vi "Close.vi"(8 "error in (no error)":errorcluster, 11 "NIScope in":refnum<class "NIScope.lvclass">) -> (0 "error out":errorcluster, 3 "NIScope out":refnum<class "NIScope.lvclass">)   [LabVIEW 2018, in "ScopePlugins.lvlib" / "NIScope.lvclass"]
doc: "Closes the connection to the scope instrument."
uses:
  NIScope.lvclass
  C:/Users/ico/Documents/Projects/NistPluggableModules/Scope/ScopePlugins/ScopePluginBaseClass/ScopePluginsBase.lvclass
  ScopePluginBaseClass/ScopePluginsBase.lvclass/ScopePluginsBase.ctl
  ScopePluginBaseClass/Accessors/Read Channels.vi
  ScopePluginBaseClass/Accessors/Write Channels.vi
  ScopePluginBaseClass/ScopePluginsBase.lvclass
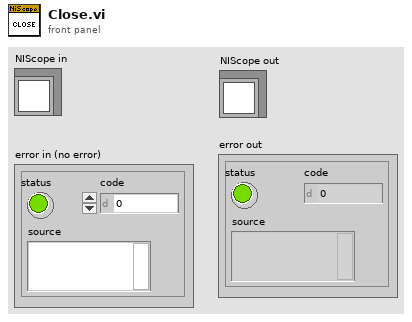
[diagram p1: front panel]
types:
  T1 = typedef "ScopePlugins.lvlib/ScopePluginsBase.lvclass/ChannelSetting(s).ctl" = cluster{"Number of Channels":i32, "Channel(s)":cluster{"Enabled":bool, "Instrument Handle":string, "Channel Name":string, "Maximum Input Frequency":dbl, "Verticle Settings":cluster{"Vertical Range":dbl, "Vertical Offset":dbl, "Probe Attenuation":dbl, "Vertical Coupling":i32}, "Connected":bool, "Input Impedance":dbl}[]}
  T2 = cluster{"Enabled":bool, "Instrument Handle":string, "Channel Name":string, "Maximum Input Frequency":dbl, "Verticle Settings":cluster{"Vertical Range":dbl, "Vertical Offset":dbl, "Probe Attenuation":dbl, "Vertical Coupling":i32}, "Connected":bool, "Input Impedance":dbl}[]
  T3 = cluster{"Enabled":bool, "Instrument Handle":string, "Channel Name":string, "Maximum Input Frequency":dbl, "Verticle Settings":cluster{"Vertical Range":dbl, "Vertical Offset":dbl, "Probe Attenuation":dbl, "Vertical Coupling":i32}, "Connected":bool, "Input Impedance":dbl}
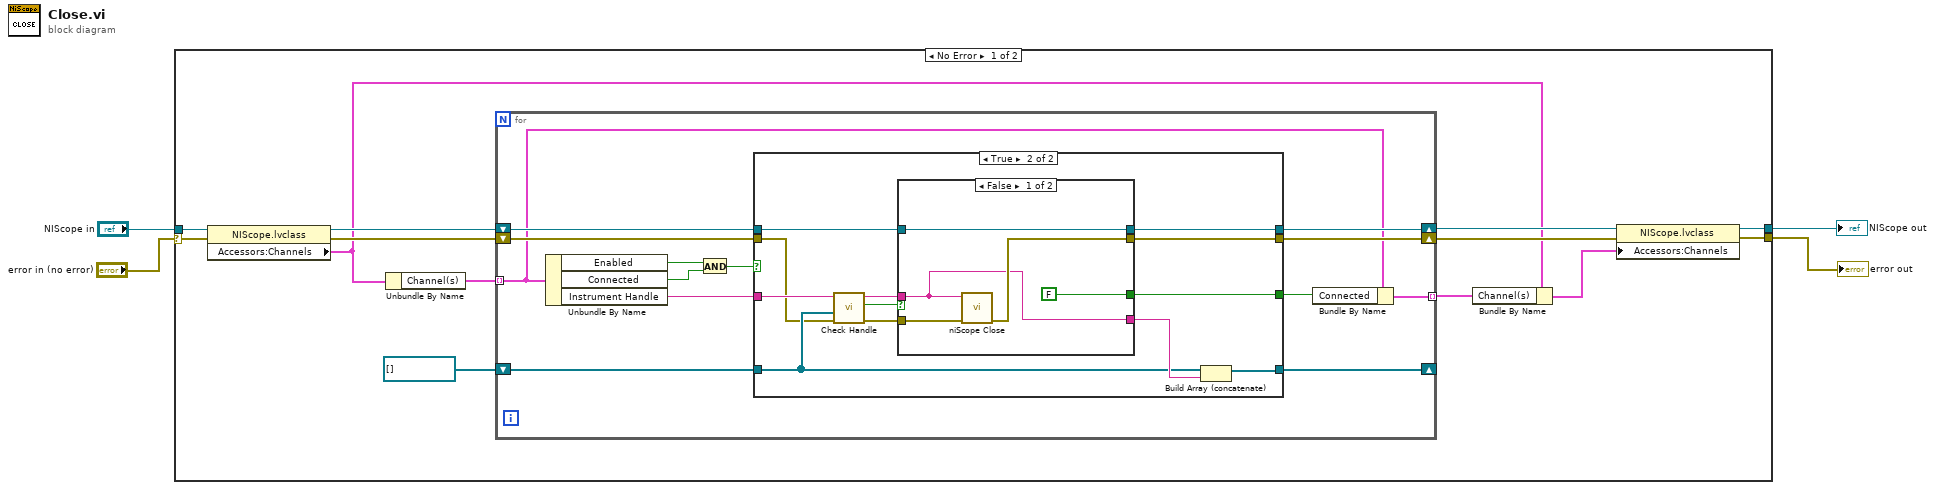
[diagram p0: block diagram]
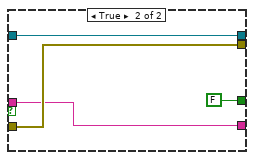
[diagram p3: hidden frame]
diagram:
  n1 = case shown="No Error" "error in (no error)" {
    selector: "error in (no error)" -> [w16 w56]
    tunnel: "NIScope in" -> [w17 w57]
    tunnel: [w11 w57] -> w2
    tunnel: [w9 w56] -> w1
    frame No Error {
      n2 = property class="NIScope.lvclass"(reference=w17, error in=w16) -> (reference out=w15:refnum<class "NIScope.lvclass">, error out=w13:errorcluster, "Accessors:Channels"=w8:T1)
      n3 = Unbundle By Name(w8) -> ("Channel(s)"=w12:T2)
      n4 = for {
        shift-right: [w26] -> w14
        shift-left: w15 -> [w30]
        shift-right: [w27] -> w10
        shift-left: w13 -> [w29]
        tunnel: w12 -> [w21] mode=indexing
        tunnel: [w24] -> w7 mode=indexing
        shift-right: [w22] -> _
        shift-left: refnum<k15>[] [] -> [w23]
        n5 = Unbundle By Name(w21) -> ("Enabled"=w19:bool, "Connected"=w18:bool, "Instrument Handle"=w28:string)
        n6 = And(x=w19, y=w18) -> (x .and. y?=w20:bool)
        n7 = case shown="True" w20 {
          selector: w20 -> [w32 _]
          tunnel: w30 -> [w34 w46]
          tunnel: w29 -> [w33 w36]
          tunnel: w28 -> [_ w38]
          tunnel: [w33 w45] -> w27
          tunnel: [w34 w44] -> w26
          tunnel: [w32 w43] -> w25
          tunnel: w23 -> [w31 w40]
          tunnel: [w31 w41] -> w22
          frame False {
          }
          frame True {
            n8 = call "Check Handle.vi"("error in (no error)"=w36, "Array"=w40, "Handle In"=w38) -> ("error out"=w35:errorcluster, "Duplicate Instrument?"=w39:bool, "Handle Out"=w37:string)  [unwired: 6 in]
            n9 = case shown="False" w39 {
              tunnel: w46 -> [w49 w55]
              tunnel: [w49 w55] -> w44
              tunnel: w35 -> [w51 w54]
              tunnel: [w50 w54] -> w45
              tunnel: [FALSE ("Connected") FALSE] -> w43
              tunnel: [w47 w52] -> w42
              tunnel: w37 -> [w47 w52]
              frame False {
                n10 = call <instrlib>:"niScope Close.vi"("instrument handle"=w47, "error in"=w51) -> ("error out"=w50:errorcluster)  [unwired: 13 in]
              }
              frame True {
              }
            }
            n11 = Build Array (concatenate)(w40, w42) -> (w41:refnum<k15>[])
          }
        }
        n12 = Bundle By Name(cluster=w21, "Connected"=w25) -> (w24:T3)
      }
      n13 = Bundle By Name(cluster=w8, "Channel(s)"=w7) -> (w6:T1)
      n14 = property class="NIScope.lvclass"(reference=w14, error in=w10, "Accessors:Channels"=w6) -> (reference out=w11:refnum<class "NIScope.lvclass">, error out=w9:errorcluster)
    }
    frame Error {
    }
  }
  "error out" <- w1
  "NIScope out" <- w2
